vi "Write_AutoGeneralOut.vi"(8 "error in (no error)":errorcluster, 10 "AutoGeneralOut":T1, 11 "AutoSubsystem in":refnum<class "AutoSubroutine.lvclass">) -> (0 "error out":errorcluster, 3 "AutoSubsystem out":refnum<class "AutoSubroutine.lvclass">)   [LabVIEW 2017, in "AutoSubroutine.lvclass"]
uses:
  AutoSubroutine.lvclass
  AutoOutput.ctl
  AutoSubroutine.lvclass/AutoSubroutine.ctl
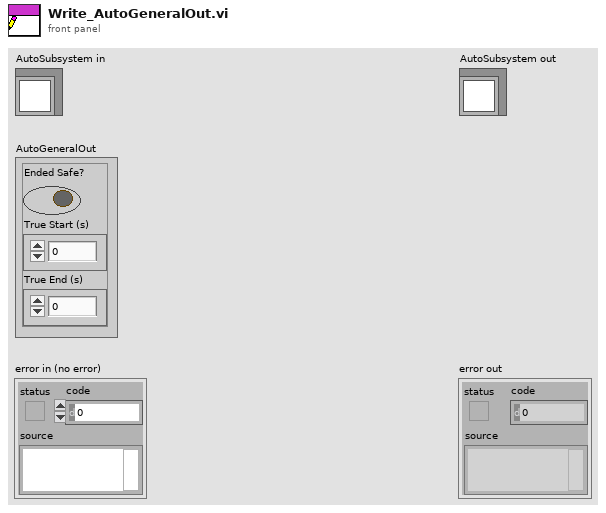
[diagram p1: front panel]
types:
  T1 = typedef "AutoSubroutine.lvclass/AutoOutput.ctl" = cluster{"Ended Safe?":bool, "True Start (s)":dbl, "True End (s)":dbl}
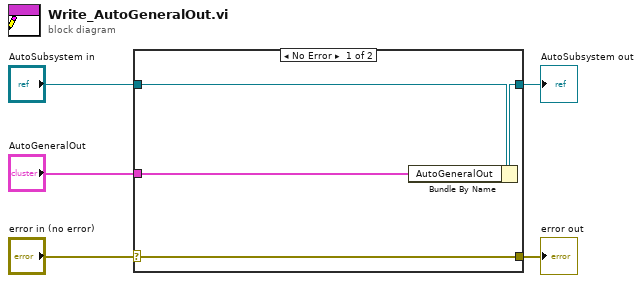
[diagram p0: block diagram]
diagram:
  n1 = case shown="No Error" "error in (no error)" {
    selector: "error in (no error)" -> [w9 w10]
    tunnel: [w9 w10] -> w4
    tunnel: [w7 w11] -> w2
    tunnel: "AutoSubsystem in" -> [w8 w11]
    tunnel: "AutoGeneralOut" -> [w6 _]
    frame No Error {
      n2 = Bundle By Name(cluster=w8, "AutoGeneralOut"=w6) -> (w7:refnum<class "AutoSubroutine.lvclass">)
    }
    frame Error {
    }
  }
  "error out" <- w4
  "AutoSubsystem out" <- w2
